vi "Power Fit Coefficients (Bisquare).vi"(0 "Y":dbl[](array[numeric]), 5 "X":dbl[](array[numeric]), 7 "Weight":dbl[](array[numeric]), 9 "tolerance":dbl=0.0001 format="%#_3g", 11 "Initial Coefficients":dbl[](array[numeric])) -> (4 "amplitude":dbl, 6 "power":dbl, 15 "error":i32)   [LabVIEW 2014, in "NI_AALPro.lvlib"]
uses:
  NI_AALPro.lvlib
  lvanlys.dll
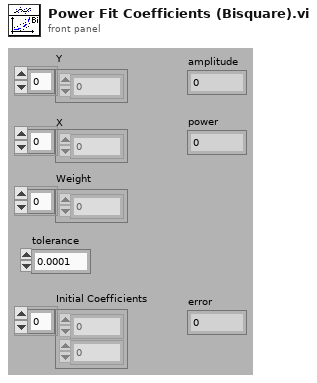
[diagram p1: front panel]
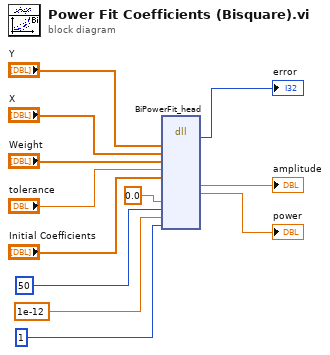
[diagram p0: block diagram]
diagram:
  n1 = dll-call lib="C:/Program Files (x86)/National Instruments/LabVIEW 2014/resource/lvanlys.*" fn="BiPowerFit_head"("y"="Y", "x"="X", "weight"="Weight", "tolerance"="tolerance", "initialCoef"="Initial Coefficients", "meanErr"=0.0, "maxIter"=50, "absTol"=1e-12, "isCoef"=1) -> (→"error":i32, "amplitude"=→"amplitude":dbl, "power"=→"power":dbl)  [unwired: 14 in, 2 out]
